vi "Show Steer Information.vi"() -> ()   [LabVIEW 2011]
uses:
  <vilib>/Rock Robotics/WPI/CAN/Jaguar/SubVIs/WPI_CANJaguar_StatusSelect.ctl
  Globals/Robot Jaguars.vi
panel:
  out "F. L. Pos":dbl
  out "F. R. Pos":dbl
  out "R. L. Pos":dbl
  out "R. R. Pos":dbl
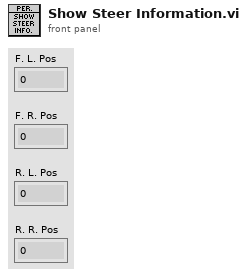
[diagram p1: front panel]
types:
  T1 = typedef "WPI_MotorControlDeviceRef.ctl" = cluster{"DeviceStatus":errorcluster, "Type":enum16{"PWM", "CAN"}, "PWM":cluster{"Digital Module":T2, "PWM Channel":T3, "DeadBand":T4}, "CAN":cluster{"Device Number":u8, "Control Mode":T5, "Semaphore":T6, "Max Vout":dbl}, "Invert":bool, "TransformRef":T7, "InvTransformRef":T7}
  T2 = typedef "FPGA_TypedefDigitalModule.ctl" = enum16{"Digital Module 1", "Digital Module 2"}
  T3 = typedef "FPGA_DIOPWMChannel.ctl" = enum8{"PWM 1", "PWM 2", "PWM 3", "PWM 4", "PWM 5", "PWM 6", "PWM 7", "PWM 8", "PWM 9", "PWM 10", "Invalid"}
  T4 = typedef "WPI_PWMDeadband.ctl" = cluster{"Name":string, "maxPositivePwm":i32, "minPositivePwm":i32, "centerPwm":i32, "maxNegativePwm":i32, "minNegativePwm":i32, "angularRange":u16}
  T5 = typedef "WPI_CANJaguar_ControlMode.ctl" = enum8{"Percent VBus", "Current", "Speed", "Position", "Voltage"}
  T6 = typedef "Semaphore RefNum" = refnum<k1>
  T7 = typedef "WPI_PWMTransform_ConPane.ctl" = refnum<vi>
  T8 = cluster{"Front Left Drive":T1, "Front Right Drive":T1, "Rear Left Drive":T1, "Rear Right Drive":T1, "Front Left Steer":T1, "Front Right Steer":T1, "Rear Left Steer":T1, "Rear Right Steer":T1}
  T9 = typedef "WPI_CANJaguar_StatusSelect.ctl" = enum16{"Output Percent VBus", "Output Voltage", "Bus Voltage", "Current", "Temperature", "Position", "Speed", "Limit Switches", "Faults", "Fault Counters", "Power Cycle"}
  T10 = typedef "WPI_CANJaguar_Status.ctl" = cluster{"Output Percent VBus":dbl, "Output Voltage":dbl, "Bus Voltage":dbl, "Current":dbl, "Temperature":dbl, "Position":dbl, "Speed":dbl, "Limits":cluster{"Forward Limit":bool, "Reverse Limit":bool, "Forward Soft Limit":bool, "Reverse Soft Limit":bool, "Sticky Forward Limit":bool, "Sticky Reverse Limit":bool, "Sticky Forward Soft Limit":bool, "Sticky Reverse Soft Limit":bool}, "Faults":cluster{"Current Fault":bool, "Temperature Fault":bool, "Bus Voltage Fault":bool, "Gate Driver Fault":bool, "Comm Fault":bool}, "Fault Counters":cluster{"Current Faults":u8, "Temperature Faults":u8, "Bus Voltage Faults":u8, "Gate Driver Faults":u8, "Comm Faults":u8, "CAN Status":u8, "CAN RX Errors":u8, "CAN TX Errors":u8}, "Power Cycle":bool}
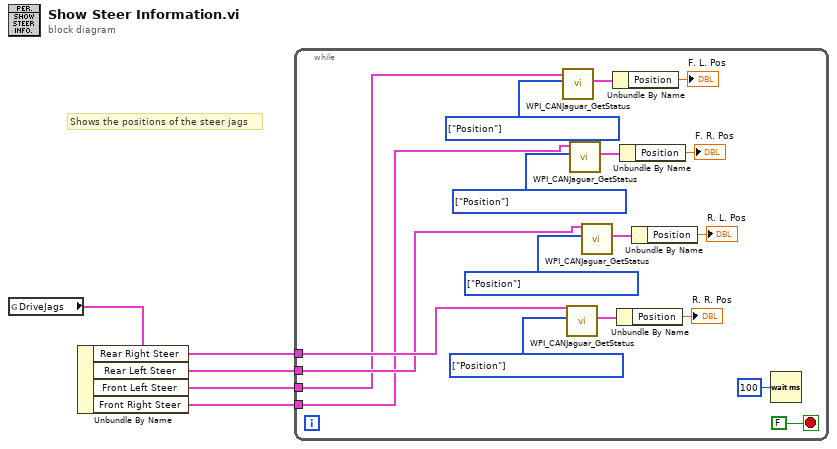
[diagram p0: block diagram]
diagram:
  # "Shows the positions of the steer jags"
  n1 = global read "Robot Jaguars.vi" "DriveJags"() -> (w1:T8)
  n2 = Unbundle By Name(w1) -> ("Rear Right Steer"=w2:T1, "Rear Left Steer"=w3:T1, "Front Left Steer"=w4:T1, "Front Right Steer"=w5:T1)
  n3 = while {
    tunnel: w2 -> [w15]
    tunnel: w3 -> [w14]
    tunnel: w4 -> [w6]
    tunnel: w5 -> [w10]
    stop <- FALSE stop-if-true
    w8 = T9[] [enum."Position"] items=["Output Percent VBus", "Output Voltage", "Bus Voltage", "Current", "Temperature", "Position", "Speed", "Limit Switches", "Faults", "Fault Counters", "Power Cycle"] ("Status Select")
    w12 = T9[] [enum."Position"] items=["Output Percent VBus", "Output Voltage", "Bus Voltage", "Current", "Temperature", "Position", "Speed", "Limit Switches", "Faults", "Fault Counters", "Power Cycle"] ("Status Select")
    w17 = T9[] [enum."Position"] items=["Output Percent VBus", "Output Voltage", "Bus Voltage", "Current", "Temperature", "Position", "Speed", "Limit Switches", "Faults", "Fault Counters", "Power Cycle"] ("Status Select")
    w20 = T9[] [enum."Position"] items=["Output Percent VBus", "Output Voltage", "Bus Voltage", "Current", "Temperature", "Position", "Speed", "Limit Switches", "Faults", "Fault Counters", "Power Cycle"] ("Status Select")
    n4 = call <vilib>:"WPI_CANJaguar_GetStatus.vi"("Status Select"=w8, "CAN Jaguar Ref"=w6) -> ("Status"=w9:T10)  [unwired: 7 in, 2 out]
    n5 = call <vilib>:"WPI_CANJaguar_GetStatus.vi"("Status Select"=w20, "CAN Jaguar Ref"=w15) -> ("Status"=w21:T10)  [unwired: 7 in, 2 out]
    n6 = call <vilib>:"WPI_CANJaguar_GetStatus.vi"("Status Select"=w12, "CAN Jaguar Ref"=w10) -> ("Status"=w11:T10)  [unwired: 7 in, 2 out]
    n7 = call <vilib>:"WPI_CANJaguar_GetStatus.vi"("Status Select"=w17, "CAN Jaguar Ref"=w14) -> ("Status"=w16:T10)  [unwired: 7 in, 2 out]
    n8 = Unbundle By Name(w9) -> ("Position"=→"F. L. Pos":dbl)
    n9 = Unbundle By Name(w21) -> ("Position"=→"R. R. Pos":dbl)
    n10 = Unbundle By Name(w11) -> ("Position"=→"F. R. Pos":dbl)
    n11 = Unbundle By Name(w16) -> ("Position"=→"R. L. Pos":dbl)
    n12 = Wait (ms)(milliseconds to wait=u32 100) -> ()  [unwired: 1 out]
  }
